vi "globalSetUp.vi"(8 "error in":errorcluster, 11 "Multiple Instances in":refnum<class "Multiple Instances.lvclass">) -> (0 "error out":errorcluster, 3 "Multiple Instances out":refnum<class "Multiple Instances.lvclass">)   [LabVIEW 2020, in "Multiple Instances.lvclass"]
uses:
  Multiple Instances.lvclass
  <vilib>/NI/VeriStand Custom Device Testing Tools/VeriStandTestUtilities/VeriStandTestUtilities.lvlib
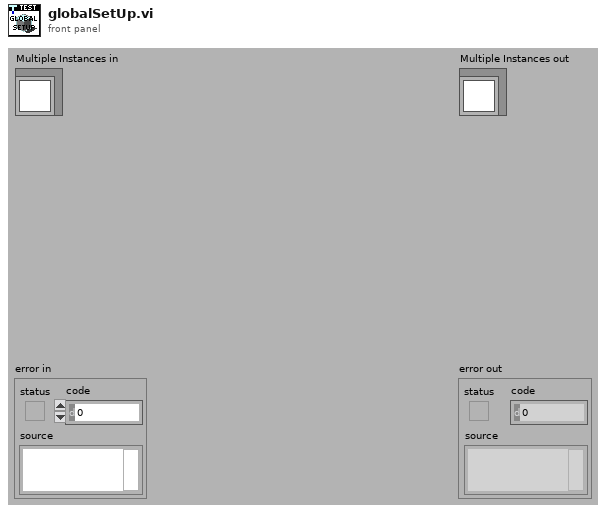
[diagram p1: front panel]
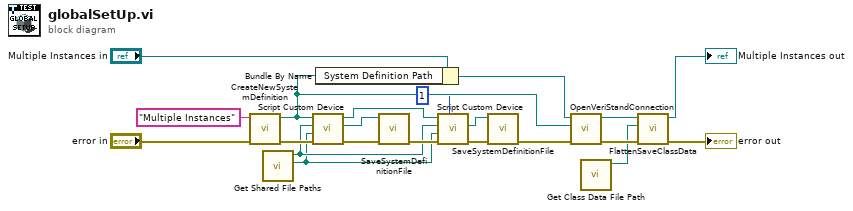
[diagram p0: block diagram]
diagram:
  n1 = call <vilib>:"CreateNewSystemDefinition.vi"("error in"="error in", "System Definition Name"="Multiple Instances") -> ("error out"=w17:errorcluster, "System Definition Path"=w13:path)  [unwired: 8 in]
  n2 = call "Get Shared File Paths.vi"() -> ("Hardware File"=w5:path, "Parameters File"=w6:path)  [unwired: 10 in]
  n3 = call "Script Custom Device.vi"("error in"=w17, "Hardware Configuration File Path"=w5, "Parameters Configuration File Path"=w6, "System Definition File Path In"=w13) -> ("error out"=w19:errorcluster, "System Definition Reference"=w18:refnum<k24>, "System Definition File Path Out"=w8:path)  [unwired: 4 in, 1 out]
  n4 = Bundle By Name(cluster="Multiple Instances in", "System Definition Path"=w13) -> (w14:refnum<class "Multiple Instances.lvclass">)
  n5 = call <vilib>:"SaveSystemDefinitionFile.vi"("error in (no error)"=w19, "System Definition Reference in"=w18) -> ("error out"=w7:errorcluster)  [unwired: 8 in, 1 out]
  n6 = call "Script Custom Device.vi"("core number"=1, "error in"=w7, "Hardware Configuration File Path"=w5, "Parameters Configuration File Path"=w6, "System Definition File Path In"=w8) -> ("error out"=w3:errorcluster, "System Definition Reference"=w2:refnum<k24>)  [unwired: 3 in, 2 out]
  n7 = call <vilib>:"SaveSystemDefinitionFile.vi"("error in (no error)"=w3, "System Definition Reference in"=w2) -> ("error out"=w1:errorcluster)  [unwired: 8 in, 1 out]
  n8 = call-dynamic "OpenVeriStandConnection.vi"("error in (no error)"=w1, "System Definition File"=w13, "VeriStand Test Case in"=w14) -> ("error out"=w15:errorcluster, "VeriStand Test Case out"=w11:refnum<class "Multiple Instances.lvclass">)  [unwired: 6 in, 1 out]
  n9 = call "Get Class Data File Path.vi"() -> ("Class Data File Path"=w12:path)  [unwired: 11 in]
  n10 = call-dynamic "FlattenSaveClassData.vi"("error in"=w15, "Class Data File Path"=w12, "VeriStandTestCase in"=w11) -> ("error out"=→"error out":errorcluster, "VeriStandTestCase out"=→"Multiple Instances out":refnum<class "Multiple Instances.lvclass">)  [unwired: 7 in]
